vi "RelayBoard_Relay_Control.vi"(8 "错误输入（无错误）":errorcluster, 9 "Relay编号":T1(ring), 10 "功能":enum16{"闭合", "断开"}(ring), 11 "端口号":refnum<visa-resource-name>="COM3" caption="VISA资源名称") -> (0 "错误输出":errorcluster)   [LabVIEW 2013]
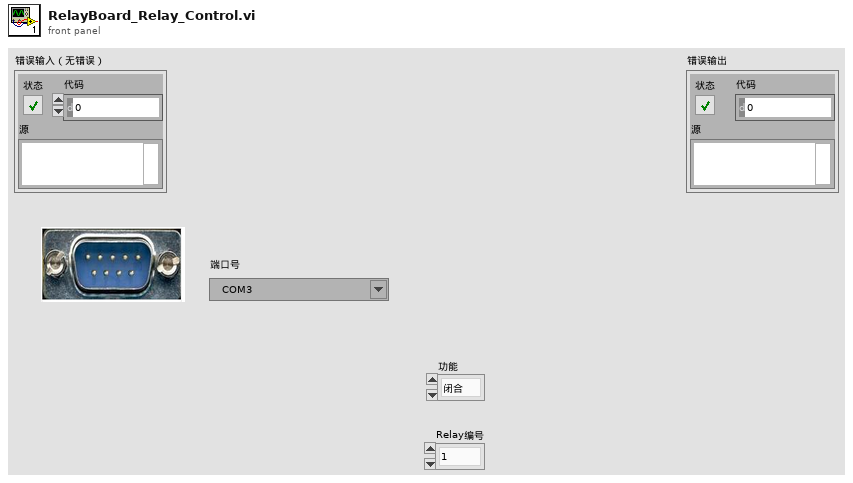
[diagram p1: front panel]
types:
  T1 = enum16{"1", "2", "3", "4", "5", "6", "7", "8", "9", "10", "11", "12", "13", "14", "15", "16"}
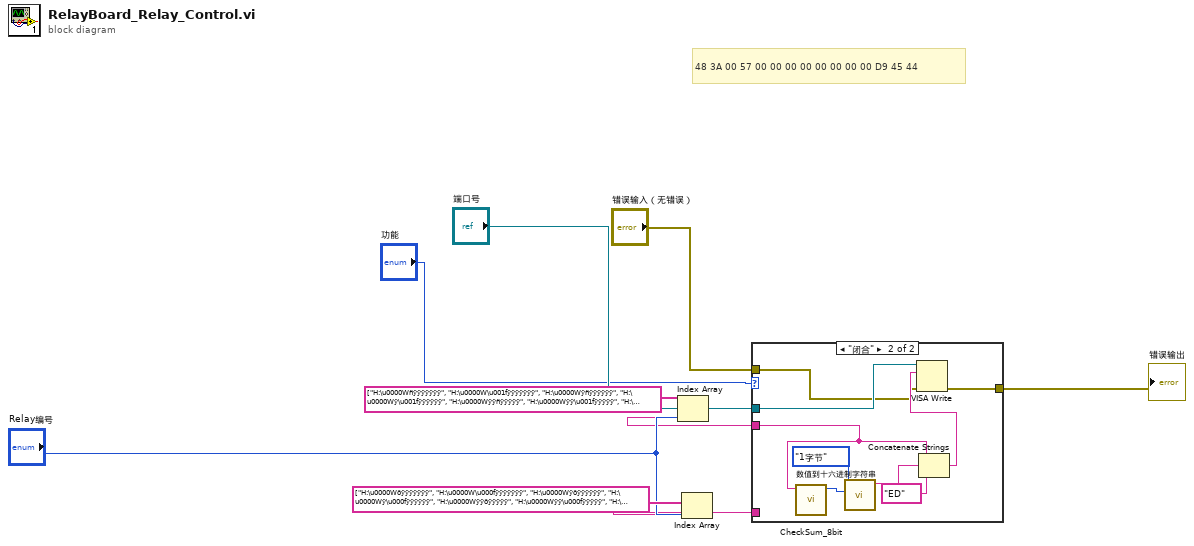
[diagram p0: block diagram]
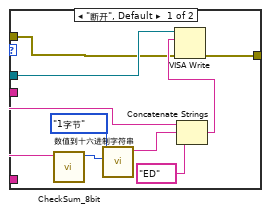
[diagram p2: hidden frame]
diagram:
  # "48 3A 00 57 00 00 00 00 00 00 00 00 D9 45 44"
  n1 = Index Array(array=string[] ["H:\u0000Wñÿÿÿÿÿÿÿ", "H:\u0000W\u001fÿÿÿÿÿÿÿ", "H:\u0000Wÿñÿÿÿÿÿÿ", "H:\u0000Wÿ\u001fÿÿÿÿÿÿ", "H:\u0000Wÿÿñÿÿÿÿÿ", "H:\u0000Wÿÿ\u001fÿÿÿÿÿ", "H:\u0000Wÿÿÿñÿÿÿÿ", "H:\u0000Wÿÿÿ\u001fÿÿÿÿ", "H:\u0000Wÿÿÿÿñÿÿÿ", "H:\u0000Wñÿÿÿ\u001fÿÿÿ", "H:\u0000Wñÿÿÿÿñÿÿ", "H:\u0000Wÿÿÿÿÿ\u001fÿÿ", "H:\u0000Wÿÿÿÿÿÿñÿ", "H:\u0000Wÿÿÿÿÿÿ\u001fÿ", "H:\u0000Wÿÿÿÿÿÿÿñ", "H:\u0000Wÿÿÿÿÿÿÿ\u001f"], index="Relay编号") -> (element=w3:string)
  n2 = Index Array(array=string[] ["H:\u0000Wðÿÿÿÿÿÿÿ", "H:\u0000W\u000fÿÿÿÿÿÿÿ", "H:\u0000Wÿðÿÿÿÿÿÿ", "H:\u0000Wÿ\u000fÿÿÿÿÿÿ", "H:\u0000Wÿÿðÿÿÿÿÿ", "H:\u0000Wÿÿ\u000fÿÿÿÿÿ", "H:\u0000Wÿÿÿðÿÿÿÿ", "H:\u0000Wÿÿÿ\u000fÿÿÿÿ", "H:\u0000Wÿÿÿÿðÿÿÿ", "H:\u0000Wñÿÿÿ\u000fÿÿÿ", "H:\u0000Wñÿÿÿÿðÿÿ", "H:\u0000Wÿÿÿÿÿ\u000fÿÿ", "H:\u0000Wÿÿÿÿÿÿðÿ", "H:\u0000Wÿÿÿÿÿÿ\u000fÿ", "H:\u0000Wÿÿÿÿÿÿÿð", "H:\u0000Wÿÿÿÿÿÿÿ\u000f"], index="Relay编号") -> (element=w4:string)
  n3 = case shown="\"闭合\"" "功能" {
    tunnel: "端口号" -> [w13 w22]
    tunnel: w4 -> [w12 _]
    tunnel: w3 -> [_ w21]
    tunnel: "错误输入（无错误）" -> [w11 w20]
    tunnel: [w10 w19] -> w1
    frame "断开", Default {
      n4 = call "CheckSum_8bit.vi"("字符串"=w12) -> ("和"=w18:u32)  [unwired: 10 in]
      n5 = call "数值到十六进制字符串.vi"("Numeric"=w18, "转换字节数"=enum16{"1字节", "2字节", "4字节", "3字节"}."1字节") -> ("转换结果"=w16:string)  [unwired: 8 in, 1 out]
      n6 = Concatenate Strings(w12, w16, "ED" ("写入缓冲区")) -> (w14:string)
      n7 = VISA Write(VISA resource name=w13, write buffer=w14, error in (no error)=w11) -> (error out=w10:errorcluster)  [unwired: 2 out]
    }
    frame "闭合" {
      n8 = call "CheckSum_8bit.vi"("字符串"=w21) -> ("和"=w27:u32)  [unwired: 10 in]
      n9 = call "数值到十六进制字符串.vi"("Numeric"=w27, "转换字节数"=enum16{"1字节", "2字节", "4字节", "3字节"}."1字节") -> ("转换结果"=w25:string)  [unwired: 8 in, 1 out]
      n10 = Concatenate Strings(w21, w25, "ED" ("写入缓冲区")) -> (w23:string)
      n11 = VISA Write(VISA resource name=w22, write buffer=w23, error in (no error)=w20) -> (error out=w19:errorcluster)  [unwired: 2 out]
    }
  }
  "错误输出" <- w1
